vi "Duplicate.vi"(8 "error in":errorcluster, 10 "parameters":variant, 11 "Fgen Instrument in":refnum<class "Fgen Instrument.lvclass">) -> (0 "error out":errorcluster, 3 "Fgen Instrument out":refnum<class "Fgen Instrument.lvclass">)   [LabVIEW 2025, in "Fgen.lvlib" / "Fgen Instrument.lvclass"]
doc: "Implements the specific behavior of a node when it is being duplicated\nCan be used to change the name of the new node for example adding Copy to it. \nCopyright 2017 National Instruments Corporation\n\nLicensed under the Apache License, Version 2.0 (the \"License\"); you may not use this file except in compliance with the License. You may obtain a copy of the License at http://www.apache.org/licenses/LICENSE-2.0\nUnless required by applicable law or agreed to in writing, software distributed under the License is distributed on an \"AS IS\" BASIS, WITHOUT WARRANTIES OR CONDITIONS OF ANY KIND, either express or implied. See the License for the specific language governing permissions and limitations under the License."
uses:
  Fgen Instrument.lvclass
  Fgen Instrument.lvclass/Fgen Instrument.ctl
  Fgen configuration/Fgen configuration.lvclass
  C:/Users/Public/Documents/Sandia National Labs/TSS Plugin/Abstract Engine.lvlibp/Instrument configuration/Instrument configuration.lvclass
  Users/Public/Documents/Sandia National Labs/TSS Plugin/Abstract Engine.lvlibp/Instrument configuration/Read Instrument Setting.vi
  Users/Public/Documents/Sandia National Labs/TSS Plugin/Abstract Engine.lvlibp/Instrument configuration/Write Instrument Setting.vi
  Users/Public/Documents/Sandia National Labs/TSS Plugin/Abstract Engine.lvlibp/Abstract Instrument/Abstract Instrument.lvclass
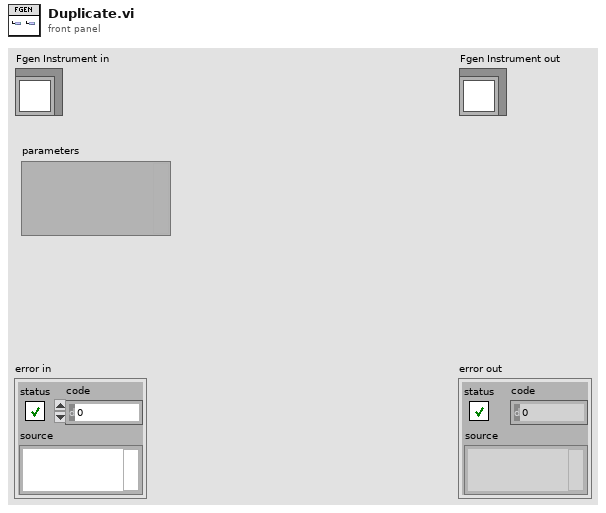
[diagram p1: front panel]
types:
  T1 = typedef "Abstract Engine.lvlibp/Instrument configuration.lvclass/Default Instrument.ctl" = cluster{"Type":string, "Address":string, "SW Alias":string, "Description":string, "Enabled":bool}
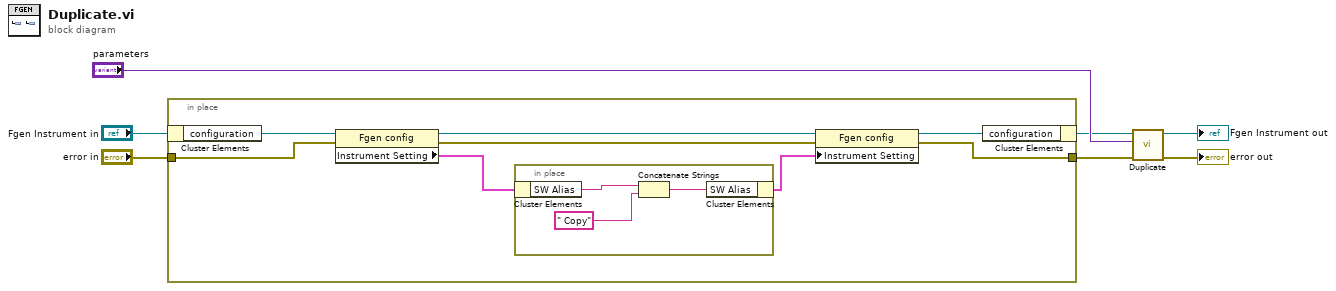
[diagram p0: block diagram]
diagram:
  n1 = in-place {
    in-place-border: "error in" -> [w15]
    in-place-border: [w13] -> w3
    n2 = in-place-cluster #1("Fgen Instrument in") -> ("configuration"=w12:refnum<class "Fgen configuration.lvclass">)
    n3 = property class="Fgen config"(reference=w12, error in=w15) -> (reference out=w9:refnum<class "Fgen configuration.lvclass">, error out=w14:errorcluster, "Instrument Setting"=w10:T1)
    n4 = in-place {
      n5 = in-place-cluster #2(w10) -> ("SW Alias"=w18:string)
      n6 = Concatenate Strings(w18, " Copy") -> (w17:string)
      n7 = in-place-cluster #2("SW Alias"=w17) -> (w8:T1)
    }
    n8 = property class="Fgen config"(reference=w9, error in=w14, "Instrument Setting"=w8) -> (reference out=w11:refnum<class "Fgen configuration.lvclass">, error out=w13:errorcluster)
    n9 = in-place-cluster #1("configuration"=w11) -> (w1:refnum<class "Fgen Instrument.lvclass">)
  }
  n10 = call-parent "Duplicate.vi"("error in"=w3, "parameters"="parameters", "CEF_Serialize node in"=w1) -> ("error out"=→"error out":errorcluster, "CEF_Serialize node out"=→"Fgen Instrument out":refnum<class "Fgen Instrument.lvclass">)  [unwired: 7 in]
